vi "Field Find In Array.vi"(9 "by DisplayName? (f, by FieldId)":bool, 10 "FieldID or Display Name(\"\")":string, 11 "Field Array":T1[](array[typedef])) -> (1 "sValue":string, 2 "Index":i32, 3 "Field":T1={"ixField"=0, "iSequenceOrder"=0, "sxFieldId"="", "sxSequenceId"="", "sDisplayName"="", "sValue"="", "sUnits"="", "nDataType"=enum."timestamp", "nNextItem"=enum."Reset", "fSystem"=FALSE, "fSystemValue"=FALSE, "fRequired"=FALSE, "fSetAtTest"=FALSE, "fTestField"=FALSE, "fDeleted"=FALSE, "fIndexed"=FALSE, "fFreeList"=FALSE})   [LabVIEW 2011]
uses:
  typedefs/Field Record.ctl
  typedefs/Field DataTypes.ctl
  typedefs/Field NextItem.ctl
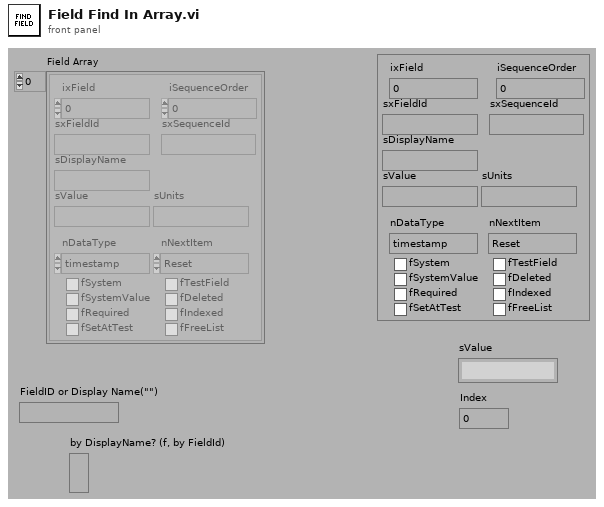
[diagram p1: front panel]
types:
  T1 = typedef "Field Record.ctl" = cluster{"ixField":i32, "iSequenceOrder":i32, "sxFieldId":string, "sxSequenceId":string, "sDisplayName":string, "sValue":string, "sUnits":string, "nDataType":T2, "nNextItem":T3, "fSystem":bool, "fSystemValue":bool, "fRequired":bool, "fSetAtTest":bool, "fTestField":bool, "fDeleted":bool, "fIndexed":bool, "fFreeList":bool}
  T2 = typedef "Field DataTypes.ctl" = enum32{"text", "numeric", "list", "timestamp", "boolean"}
  T3 = typedef "Field NextItem.ctl" = enum32{"Reset", "Retain", "Auto-Increment"}
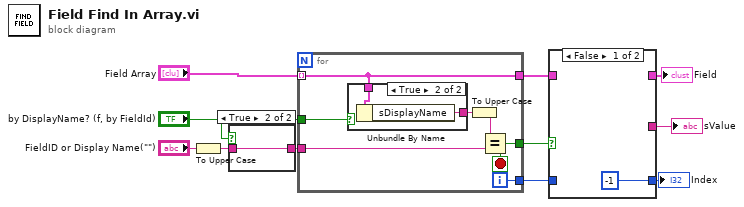
[diagram p0: block diagram]
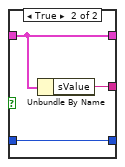
[diagram p2: hidden frame]
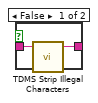
[diagram p3: hidden frame]
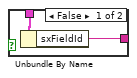
[diagram p4: hidden frame]
diagram:
  n1 = To Upper Case(1:"FieldID or Display Name(\"\")") -> (0:w8:string)
  n2 = case shown="True" "by DisplayName? (f, by FieldId)" {
    tunnel: w8 -> [w13 w14]
    tunnel: [w12 w14] -> w7
    frame False {
      n3 = call "TDMS Strip Illegal Characters.vi"("String"=w13) -> ("Legal String"=w12:string)  [unwired: 4 out]
    }
    frame True {
    }
  }
  n4 = for {
    tunnel: "Field Array" -> [w21] mode=indexing
    tunnel: w7 -> [w20]
    tunnel: [w16] -> w6
    tunnel: [w21] -> w5
    tunnel: "by DisplayName? (f, by FieldId)" -> [w17]
    tunnel: [w15] -> w4
    i -> [w15]
    stop <- w16 stop-if-true
    n5 = case shown="True" w17 {
      tunnel: w21 -> [w23 w25]
      tunnel: [w22 w24] -> w19
      frame False {
        n6 = Unbundle By Name(w23) -> ("sxFieldId"=w22:string)
      }
      frame True {
        n7 = Unbundle By Name(w25) -> ("sDisplayName"=w24:string)
      }
    }
    n8 = To Upper Case(1:w19) -> (0:w18:string)
    n9 = Equal?(x=w18, y=w20) -> (x = y?=w16:bool)
  }
  n10 = case shown="False" w6 {
    tunnel: w5 -> [_ w28]
    tunnel: w4 -> [_ w29]
    tunnel: [_ w28] -> w3
    tunnel: [-1 w29] -> w2
    tunnel: [_ w27] -> w1
    frame False {
    }
    frame True {
      n11 = Unbundle By Name(w28) -> ("sValue"=w27:string)
    }
  }
  "Field" <- w3
  "Index" <- w2
  "sValue" <- w1
